vi "Write AO Line.vi"(7 "AO line":T1=5100 items=["ModB/AO0"=5100, "ModB/AO1"=5101, "ModB/AO2"=5102, "ModB/AO3"=5103], 8 "error in (no error)":errorcluster, 10 "data":dbl, 11 "starter kit host in":refnum<class "NI_Robotics_Starter Kit Host.lvclass">) -> (0 "error out":errorcluster, 3 "starter kit host out":refnum<class "NI_Robotics_Starter Kit Host.lvclass">)   [LabVIEW 2017, in "NI_Robotics_Starter Kit Host.lvclass"]
doc: "Writes a voltage value to an analog output line on the Starter Kit FPGA."
uses:
  <vilib>/robotics/Starter Kit/Host Interface/NI_Robotics_Starter Kit Host.lvclass
  <vilib>/robotics/Starter Kit/Direct IO/AO Lines.ctl
  <vilib>/robotics/Starter Kit/Host Interface/NI_Robotics_Starter Kit Host.lvclass/NI_Robotics_Starter Kit Host.ctl
  <vilib>/robotics/Utilities/Generate Error.vi
  <vilib>/robotics/Starter Kit/Direct IO/NI_Robotics_Starter Kit Direct IO.lvclass
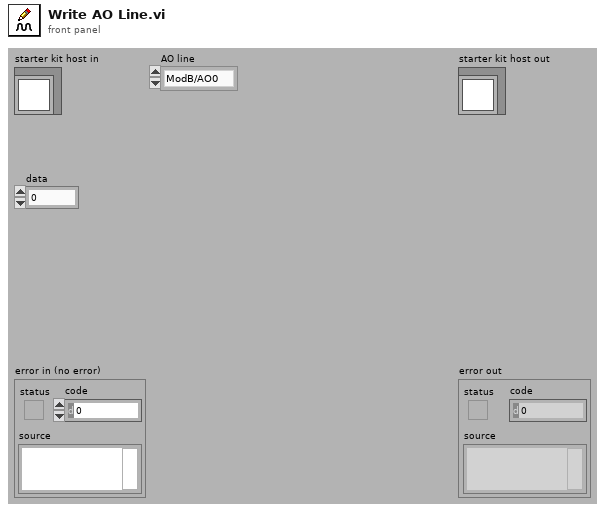
[diagram p1: front panel]
types:
  T1 = typedef "NI_Robotics_Starter Kit Direct IO.lvclass/AO Lines.ctl" = u16
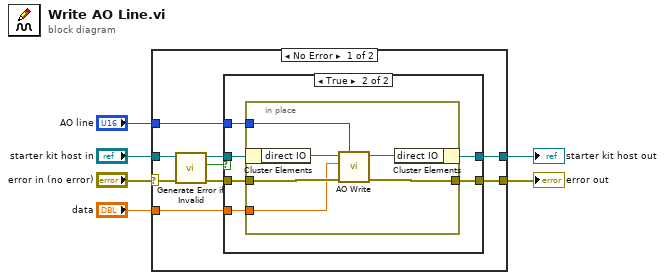
[diagram p0: block diagram]
diagram:
  n1 = case shown="No Error" "error in (no error)" {
    selector: "error in (no error)" -> [w9 w31]
    tunnel: [w13 w31] -> w3
    tunnel: [w15 w30] -> w2
    tunnel: "starter kit host in" -> [w11 w30]
    tunnel: "AO line" -> [w14 _]
    tunnel: "data" -> [w12 _]
    frame No Error {
      n2 = call <vilib>:"Generate Error if Invalid.vi"("error in (no error)"=w9, "starter kit host in"=w11) -> ("error out"=w8:errorcluster, "valid?"=w7:bool, "starter kit host out"=w10:refnum<class "NI_Robotics_Starter Kit Host.lvclass">)  [unwired: 7 in]
      n3 = case shown="True" w7 {
        tunnel: [w17 w23] -> w15
        tunnel: w14 -> [_ w22]
        tunnel: [w16 w21] -> w13
        tunnel: w12 -> [_ w20]
        tunnel: w10 -> [w17 w19]
        tunnel: w8 -> [w16 w18]
        frame False {
        }
        frame True {
          n4 = in-place {
            in-place-border: w18 -> [w26]
            in-place-border: [w25] -> w21
            in-place-border: w22 -> [w27]
            in-place-border: w20 -> [w24]
            n5 = in-place-cluster #1(w19) -> ("direct IO"=w29:refnum<class "NI_Robotics_Starter Kit Direct IO.lvclass">)
            n6 = call-dynamic "AO Write.vi"("AO line"=w27, "error in (no error)"=w26, "data"=w24, "direct IO in"=w29) -> ("error out"=w25:errorcluster, "direct IO out"=w28:refnum<class "NI_Robotics_Starter Kit Direct IO.lvclass">)  [unwired: 6 in]
            n7 = in-place-cluster #1("direct IO"=w28) -> (w23:refnum<class "NI_Robotics_Starter Kit Host.lvclass">)
          }
        }
      }
    }
    frame Error {
    }
  }
  "error out" <- w3
  "starter kit host out" <- w2
